vi "TLC Main (Classes).vi"(8 "error in (no error)":errorcluster) -> (0 "error out":errorcluster)   [LabVIEW 2010]
doc: "This version of TLC Main.vi uses LabVIEW classes to define the different application commands that are sent from the producer to the consumer loop. Instead of enqueueing a command and a variant which must be converted, a generic Application Command class is defined and child classes are defined for each function to be performed by the consumer loop. \n\nThis removes the need for extracting and converting the variant data and implementing separate cases for each command. That method is still used in the display loop. Compare and contrast the two methods of handling abstraction of data (variants vs classes)."
uses:
  Controls/tlc_Cue_Information.ctl
  Controls/channel.ctl
  Application Command/Application Command.lvclass
  Controls/tlc_User Interface Command.ctl
  Controls/tlc_User Interface Data Type.ctl
  Modules/Cue/tlc_Cue_Information Command.ctl
  Exit/Exit App.lvclass
  Record/Record.lvclass
  Save/Save.lvclass
  Load/Load.lvclass
  Stop/Stop.lvclass
  Play/Play.lvclass
  Initialize Application/Initialize Application.lvclass
panel:
  out "Cue Information":T1 {"Channels"."Intensity" min=0.0 max=100.0 step=1.0 format="%#.0f"}
  in  "Stop":bool
  in  "Record":bool
  in  "Play":bool
  out "Cue List":i32(listbox)
  # "Cue Control"
  # "Cue Information"
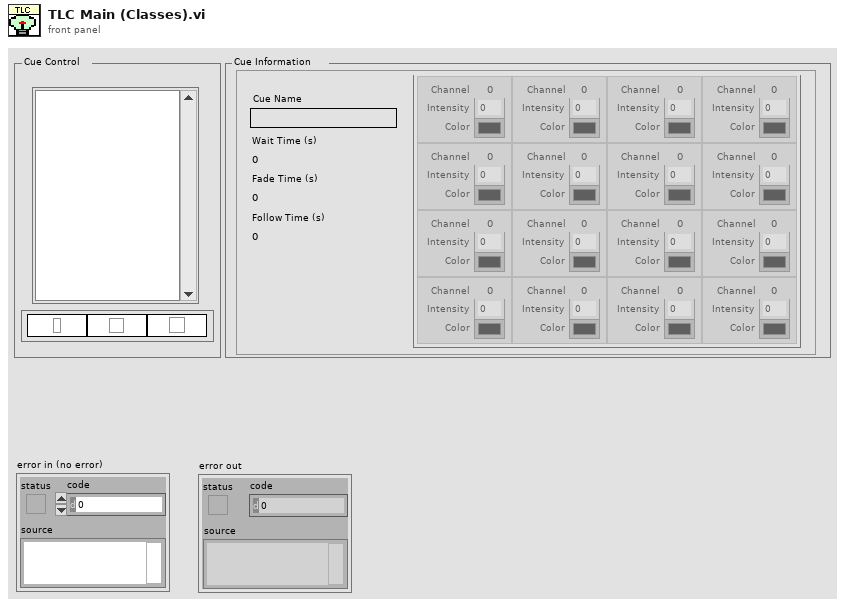
[diagram p1: front panel]
types:
  T1 = typedef "tlc_Cue_Information.ctl" = cluster{"Cue Name":string, "Wait Time (s)":u32, "Fade Time (s)":u32, "Follow Time (s)":u32, "Channels":T2[][]}
  T2 = typedef "channel.ctl" = cluster{"Intensity":dbl, " Color":u32, "Channel":i32}
  T3 = typedef "tlc_User Interface Command.ctl" = cluster{"Data Type":T4, "Data":variant}
  T4 = typedef "tlc_User Interface Data Type.ctl" = enum16{"Initialize", "Initialize Front Panel", "Update Front Panel Channels", "Select Cue in Cue List", "Enable/Disable Front Panel Controls", "Update Cue List", "Stop"}
  T5 = typedef "tlc_Cue_Information Command.ctl" = enum16{"Add Cue", "Get Cue Values", "Set Cue Values", "Get Number of Cues", "Initialize", "Get Empty Cue"}
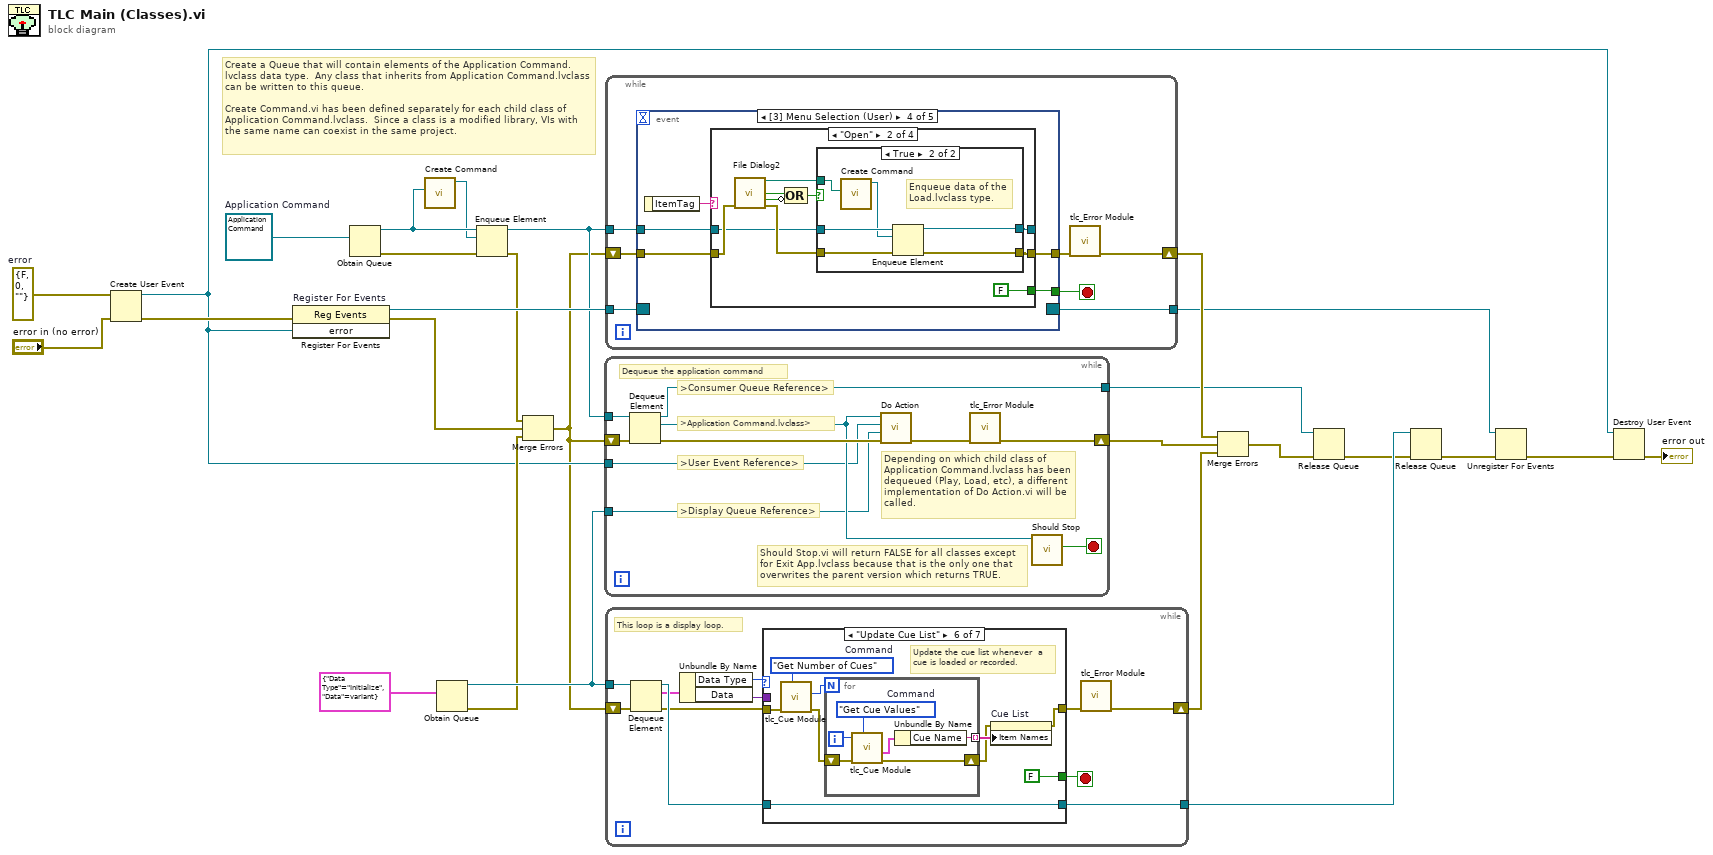
[diagram p0: block diagram]
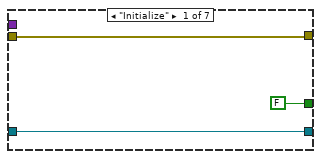
[diagram p2: hidden frame]
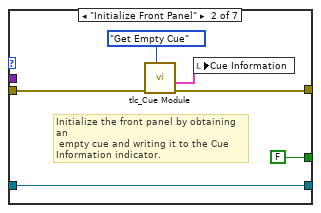
[diagram p3: hidden frame]
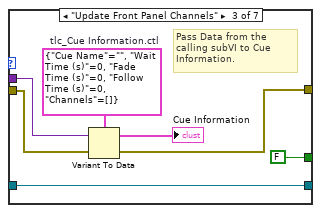
[diagram p4: hidden frame]
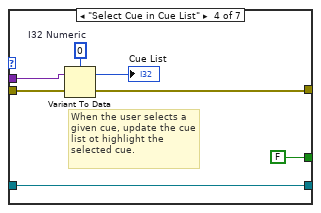
[diagram p5: hidden frame]
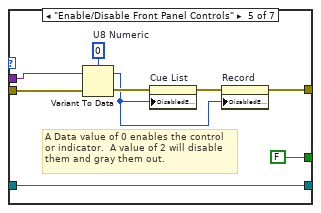
[diagram p6: hidden frame]
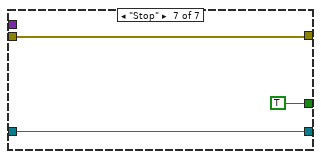
[diagram p7: hidden frame]
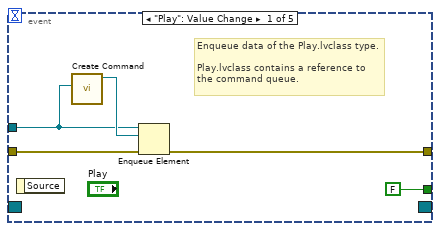
[diagram p8: hidden frame]
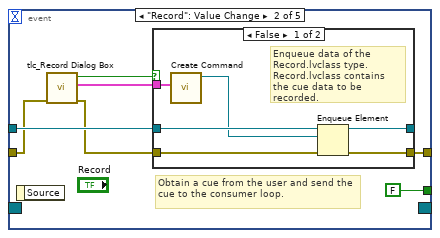
[diagram p9: hidden frame]
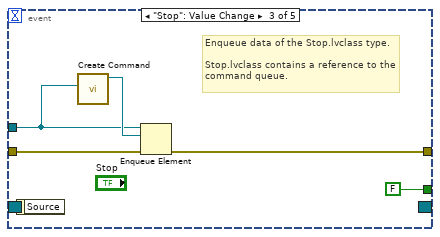
[diagram p11: hidden frame]
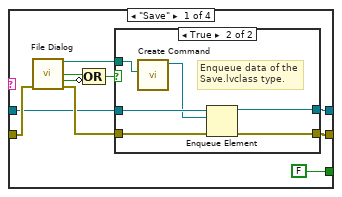
[diagram p12: hidden frame]
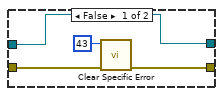
[diagram p13: hidden frame]
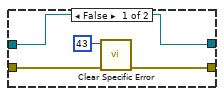
[diagram p14: hidden frame]
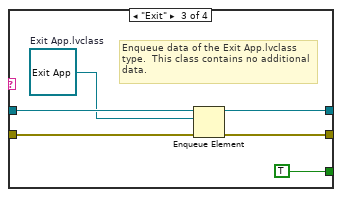
[diagram p15: hidden frame]
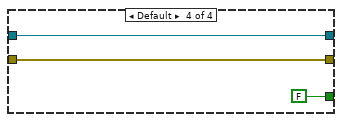
[diagram p16: hidden frame]
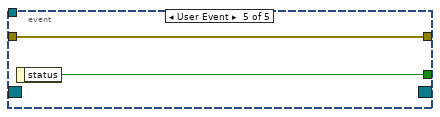
[diagram p17: hidden frame]
diagram:
  w26 = errorcluster {"status"=FALSE, "code"=0, "source"=""}  # error
  w27 = refnum<class "Application Command.lvclass"> refnum  # Application Command
  # "Create a Queue that will contain elements of the Application Command.lvclass data type.  Any class that inherits from Application Command.lvclass can be written to this queue.\n\nCreate Command.vi has been defined separately for each child class of Application Command.lvclass.  Since a class is a modified library, VIs with the same name can coexist in the same project."
  n1 = Create User Event(user event datatype=w26, error in="error in (no error)") -> (user event=w9:refnum<user-event>, error out=w25:errorcluster)
  n2 = register-events "Register For Events"(error in=w25, w9) -> (reference out=w24:refnum<event-registration>, error out=w13:errorcluster)  [unwired: 1 in]
  n3 = Obtain Queue(element data type=w27) -> (queue out=w3:refnum<queue>, error out=w6:errorcluster)  [unwired: 4 in, 1 out]
  n4 = call "Create Command.vi"("Command Queue"=w3) -> ("Initialize Application.lvclass"=w2:refnum<class "Initialize Application.lvclass">)  [unwired: 10 in]
  n5 = Obtain Queue(element data type=T3 {"Data Type"=enum."Initialize", "Data"=variant} ("tlc_User Interface Command.ctl")) -> (queue out=w11:refnum<queue>, error out=w10:errorcluster)  [unwired: 4 in, 1 out]
  n6 = Enqueue Element(queue=w3, element=w2, error in (no error)=w6) -> (queue out=w5:refnum<queue>, error out=w4:errorcluster)  [unwired: 1 in, 1 out]
  n7 = Merge Errors(w4, w13, w10) -> (w1:errorcluster)
  n8 = while {
    shift-right: [w30] -> w8
    shift-left: w1 -> [w36]
    tunnel: w5 -> [w37]
    tunnel: [w34] -> w21
    tunnel: w11 -> [w31]
    tunnel: w9 -> [w29]
    stop <- w33 stop-if-true
    # "Should Stop.vi will return FALSE for all classes except for Exit App.lvclass because that is the only one that overwrites the parent version which returns TRUE."
    # "Depending on which child class of Application Command.lvclass has been dequeued (Play, Load, etc), a different implementation of Do Action.vi will be called."
    # "Dequeue the application command"
    # ">Consumer Queue Reference>"
    # ">Application Command.lvclass>"
    # ">Display Queue Reference>"
    # ">User Event Reference>"
    n9 = Dequeue Element(queue=w37, error in (no error)=w36) -> (queue out=w34:refnum<queue>, element=w32:refnum<class "Application Command.lvclass">, error out=w35:errorcluster)  [unwired: 1 in, 1 out]
    n10 = call-dynamic "Do Action.vi"("error in (no error)"=w35, "Display Queue"=w31, "tlc_User Event Reference.ctl"=w29, "Application Command in"=w32) -> ("error out"=w28:errorcluster)  [unwired: 7 in]
    n11 = call "tlc_Error Module.vi"("error in (no error)"=w28) -> ("error out"=w30:errorcluster)  [unwired: 9 in, 1 out]
    n12 = call-dynamic "Should Stop.vi"("Application Command.lvclass"=w32) -> ("stop?"=w33:bool)  [unwired: 10 in]
  }
  n13 = while {
    shift-right: [w38] -> w22
    shift-left: w1 -> [w43]
    tunnel: w24 -> [w41]
    tunnel: [w40] -> w20
    tunnel: w5 -> [w44]
    stop <- w42 stop-if-true
    n14 = event shown="[3] Menu Selection (User)" {
      selector: w41 -> [_ _ _ _ _]
      dyn-events: [_ _ _ _ _] -> w40
      timeout: _ -> [_ _ _ _ _]
      tunnel: w44 -> [w45 w55 w65 w73 _]
      tunnel: w43 -> [w48 w53 w68 w72 w124]
      tunnel: [w47 w54 w67 w71 w124] -> w39
      tunnel: [FALSE FALSE FALSE w70 w125] -> w42
      event "Play": Value Change {
        # "Enqueue data of the Play.lvclass type.  \n\nPlay.lvclass contains a reference to the command queue."
        n15 = event-data() -> ()  [unwired: 1 in, 1 out]
        n16 = call "Create Command.vi"("Command Queue"=w45) -> ("Play.lvclass"=w46:refnum<class "Play.lvclass">)  [unwired: 10 in]
        n17 = Enqueue Element(queue=w45, element=w46, error in (no error)=w48) -> (error out=w47:errorcluster)  [unwired: 1 in, 2 out]
      }
      event "Record": Value Change {
        # "Obtain a cue from the user and send the cue to the consumer loop."
        n18 = event-data() -> ()  [unwired: 1 in, 1 out]
        n19 = call "tlc_Record Dialog Box.vi"("error in (no error)"=w53) -> ("error out"=w52:errorcluster, "Output Cue"=w50:T1, "Cancelled?"=w51:bool)  [unwired: 8 in]
        n20 = case shown="False" w51 {
          tunnel: w55 -> [w62 w64]
          tunnel: w52 -> [w61 w63]
          tunnel: [w60 w63] -> w54
          tunnel: [w59 w64] -> _
          tunnel: w50 -> [w58 _]
          frame False {
            # "Enqueue data of the Record.lvclass type.  \nRecord.lvclass contains the cue data to be recorded."
            n21 = call "Create Command.vi"("Cue Information"=w58) -> ("Record out"=w57:refnum<class "Record.lvclass">)  [unwired: 10 in]
            n22 = Enqueue Element(queue=w62, element=w57, error in (no error)=w61) -> (queue out=w59:refnum<queue>, error out=w60:errorcluster)  [unwired: 1 in, 1 out]
          }
          frame True {
          }
        }
      }
      event "Stop": Value Change {
        # "Enqueue data of the Stop.lvclass type.  \n\nStop.lvclass contains a reference to the command queue."
        n23 = event-data() -> ()  [unwired: 1 in, 1 out]
        n24 = call "Create Command.vi"("Command Queue"=w65) -> ("Stop.lvclass"=w66:refnum<class "Stop.lvclass">)  [unwired: 10 in]
        n25 = Enqueue Element(queue=w65, element=w66, error in (no error)=w68) -> (error out=w67:errorcluster)  [unwired: 1 in, 2 out]
      }
      event Menu Selection (User) {
        n26 = event-data() -> ("ItemTag"=w74:string)  [unwired: 1 in]
        n27 = case shown="\"Open\"" w74 {
          tunnel: w73 -> [w75 w95 w120 w123]
          tunnel: w72 -> [w83 w103 w118 w122]
          tunnel: [w79 w99 w119 w123] -> _
          tunnel: [w80 w100 w117 w122] -> w71
          tunnel: [FALSE FALSE TRUE FALSE] -> w70
          frame "Save" {
            n28 = call "File Dialog"("error in"=w83) -> ("selected path"=w76:path, "exists"=w82:bool, "cancelled"=w81:bool, "error out"=w78:errorcluster)  [unwired: 11 in]
            n29 = Compound Arithmetic op=OR(w82, invert w81) -> (w77:bool)
            n30 = case shown="True" w77 {
              tunnel: [w87 w94] -> w80
              tunnel: [w85 w93] -> w79
              tunnel: w78 -> [w88 w92]
              tunnel: w76 -> [_ w90]
              tunnel: w75 -> [w85 w91]
              frame False {
                n31 = call "Clear Specific Error.vi"("error in (no error)"=w88, "Code"=43) -> ("error out"=w87:errorcluster)  [unwired: 5 in]
              }
              frame True {
                # "Enqueue data of the Save.lvclass type."
                n32 = call "Create Command.vi"("Save Path"=w90) -> ("Save.lvclass"=w89:refnum<class "Save.lvclass">)  [unwired: 10 in]
                n33 = Enqueue Element(queue=w91, element=w89, error in (no error)=w92) -> (queue out=w93:refnum<queue>, error out=w94:errorcluster)  [unwired: 1 in, 1 out]
              }
            }
          }
          frame "Open" {
            n34 = call "File Dialog2"("error in"=w103) -> ("selected path"=w96:path, "exists"=w102:bool, "cancelled"=w101:bool, "error out"=w98:errorcluster)  [unwired: 11 in]
            n35 = Compound Arithmetic op=OR(w102, invert w101) -> (w97:bool)
            n36 = case shown="True" w97 {
              tunnel: [w107 w114] -> w100
              tunnel: [w105 w113] -> w99
              tunnel: w98 -> [w108 w112]
              tunnel: w96 -> [_ w110]
              tunnel: w95 -> [w105 w111]
              frame False {
                n37 = call "Clear Specific Error.vi"("error in (no error)"=w108, "Code"=43) -> ("error out"=w107:errorcluster)  [unwired: 5 in]
              }
              frame True {
                # "Enqueue data of the Load.lvclass type."
                n38 = call "Create Command.vi"("Path to file"=w110) -> ("Load.lvclass"=w109:refnum<class "Load.lvclass">)  [unwired: 10 in]
                n39 = Enqueue Element(queue=w111, element=w109, error in (no error)=w112) -> (queue out=w113:refnum<queue>, error out=w114:errorcluster)  [unwired: 1 in, 1 out]
              }
            }
          }
          frame "Exit" {
            w115 = refnum<class "Exit App.lvclass"> refnum  # Exit App.lvclass
            # "Enqueue data of the Exit App.lvclass type.  This class contains no additional data."
            n40 = Enqueue Element(queue=w120, element=w115, error in (no error)=w118) -> (queue out=w119:refnum<queue>, error out=w117:errorcluster)  [unwired: 1 in, 1 out]
          }
          frame Default {
          }
        }
      }
      event User Event {
        n41 = event-data() -> ("status"=w125:bool)  [unwired: 1 in]
      }
    }
    n42 = call "tlc_Error Module.vi"("error in (no error)"=w39) -> ("error out"=w38:errorcluster)  [unwired: 9 in, 1 out]
  }
  n43 = while {
    shift-right: [w126] -> w14
    shift-left: w1 -> [w134]
    tunnel: [w135] -> w15
    tunnel: w11 -> [w129]
    stop <- w131 stop-if-true
    # "This loop is a display loop."
    n44 = Dequeue Element(queue=w129, error in (no error)=w134) -> (queue out=w136:refnum<queue>, element=w133:T3, error out=w132:errorcluster)  [unwired: 1 in, 1 out]
    n45 = Unbundle By Name(w133) -> ("Data Type"=w128:T4, "Data"=w130:variant)
    n46 = case shown="\"Update Cue List\"" w128 {
      tunnel: w136 -> [w138 w145 w152 w159 w168 w177 w185]
      tunnel: [w138 w145 w152 w159 w168 w177 w185] -> w135
      tunnel: w132 -> [w139 w142 w150 w157 w166 w175 w186]
      tunnel: [w139 w141 w148 w155 w161 w173 w186] -> w127
      tunnel: [FALSE FALSE FALSE FALSE FALSE FALSE TRUE] -> w131
      tunnel: w130 -> [_ _ w149 w156 w165 _ _]
      frame "Initialize" {
      }
      frame "Initialize Front Panel" {
        # "Initialize the front panel by obtaining an\n empty cue and writing it to the Cue Information indicator."
        n47 = call "tlc_Cue Module.vi"("Command"=tlc_Cue_Information_Command."Get Empty Cue", "error in (no error)"=w142) -> ("error out"=w141:errorcluster, "Cue Output"=w140:T1)  [unwired: 6 in, 1 out]
        n48 = local write "Cue Information"(w140) -> ()
      }
      frame "Update Front Panel Channels" {
        w146 = T1 {"Cue Name"="", "Wait Time (s)"=0, "Fade Time (s)"=0, "Follow Time (s)"=0, "Channels"=[]}  # tlc_Cue Information.ctl
        # "Pass Data from the calling subVI to Cue Information."
        n49 = Variant To Data(error in=w150, Variant=w149, type=w146) -> (error out=w148:errorcluster, data=→"Cue Information":T1)
      }
      frame "Select Cue in Cue List" {
        w153 = 0  # I32 Numeric
        # "When the user selects a given cue, update the cue list ot highlight the selected cue."
        n50 = Variant To Data(error in=w157, Variant=w156, type=w153) -> (error out=w155:errorcluster, data=→"Cue List":i32)
      }
      frame "Enable/Disable Front Panel Controls" {
        w164 = 0  # U8 Numeric
        # "A Data value of 0 enables the control or indicator.  A value of 2 will disable them and gray them out."
        n51 = Variant To Data(error in=w166, Variant=w165, type=w164) -> (error out=w163:errorcluster, data=w160:i32)
        n52 = property on="Cue List" class="LstBox (strict)"(error in=w163, "DisabledEnum"=w160) -> (error out=w162:errorcluster)  [unwired: 1 in, 1 out]
        n53 = property on="Record" class="Bool"(error in=w162, "DisabledEnum"=w160) -> (error out=w161:errorcluster)  [unwired: 1 in, 1 out]
      }
      frame "Update Cue List" {
        w174 = tlc_Cue_Information_Command."Get Number of Cues"  # Command
        # "Update the cue list whenever  a cue is loaded or recorded."
        n54 = call "tlc_Cue Module.vi"("Command"=w174, "error in (no error)"=w175) -> ("error out"=w170:errorcluster, "Number of Cues"=w172:i32)  [unwired: 6 in, 1 out]
        n55 = for {
          N: w172 -> [_]
          tunnel: [w180] -> w171 mode=indexing
          shift-right: [w179] -> w169
          shift-left: w170 -> [w178]
          i -> [w182]
          w183 = tlc_Cue_Information_Command."Get Cue Values"  # Command
          n56 = call "tlc_Cue Module.vi"("Command"=w183, "error in (no error)"=w178, "Cue Index"=w182) -> ("error out"=w179:errorcluster, "Cue Output"=w181:T1)  [unwired: 5 in, 1 out]
          n57 = Unbundle By Name(w181) -> ("Cue Name"=w180:string)
        }
        n58 = property on="Cue List" class="LstBox (strict)"(error in=w169, "Item Names"=w171) -> (error out=w173:errorcluster)  [unwired: 1 in, 1 out]
      }
      frame "Stop" {
      }
    }
    n59 = call "tlc_Error Module.vi"("error in (no error)"=w127) -> ("error out"=w126:errorcluster)  [unwired: 9 in, 1 out]
  }
  n60 = Merge Errors(w22, w8, w14) -> (w12:errorcluster)
  n61 = Release Queue(queue=w21, error in (no error)=w12) -> (error out=w7:errorcluster)  [unwired: 1 in, 2 out]
  n62 = Release Queue(queue=w15, error in (no error)=w7) -> (error out=w16:errorcluster)  [unwired: 1 in, 2 out]
  n63 = Unregister For Events(event registration refnum=w20, error in=w16) -> (error out=w19:errorcluster)
  n64 = Destroy User Event(user event=w9, error in=w19) -> (error out=→"error out":errorcluster)
